vi "exec.vi"(8 "error in (no error)":errorcluster, 10 "context":refnum<class "Context.lvclass">, 11 "ForceSetpoint in":refnum<class "ForceSetpoint.lvclass">) -> (0 "error out":errorcluster, 2 "context 2":refnum<class "Context.lvclass">, 3 "ForceSetpoint out":refnum<class "ForceSetpoint.lvclass">)   [LabVIEW 2013, in "ForceSetpoint.lvclass"]
uses:
  ForceSetpoint.lvclass
  Context/Context.lvclass
  ForceSetpoint.lvclass/ForceSetpoint.ctl
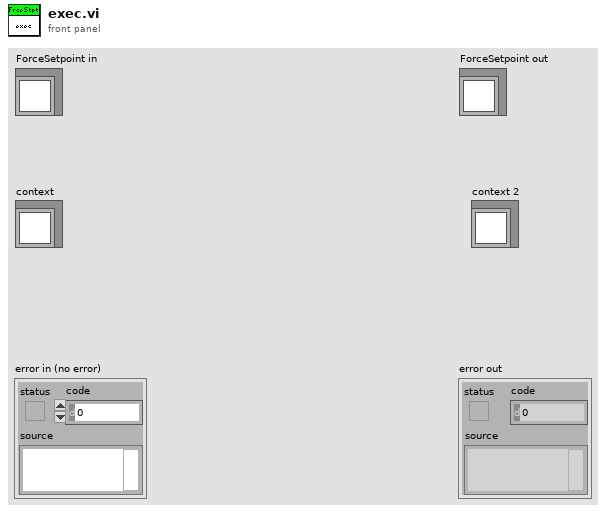
[diagram p1: front panel]
types:
  T1 = typedef "FAMTTypedefs.lvlib/ForceSetpoint.ctl" = dbl[unit]
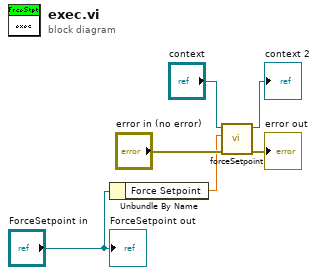
[diagram p0: block diagram]
diagram:
  n1 = Unbundle By Name("ForceSetpoint in") -> ("Force Setpoint"=w1:T1)
  n2 = call "forceSetpoint.vi"("error in (no error)"="error in (no error)", "Force Setpoint"=w1, "Context in"="context") -> ("error out"=→"error out":errorcluster, "Context out"=→"context 2":refnum<class "Context.lvclass">)  [unwired: 7 in]
  "ForceSetpoint out" <- "ForceSetpoint in"
